vi "solar_qtimer Get Qtimer Names for Target.vi"(10 "Target Name":string, 11 "QTimers":T1[](array[typedef])) -> (3 "Target's Qtimer Names":string[](array[string]))   [LabVIEW 2018]
doc: "Outputs target names for each of the specified qtimers."
uses:
  solar_qtimer_ctl QTimer Settings.ctl
  solar_qtimer_ctl QTimer.ctl
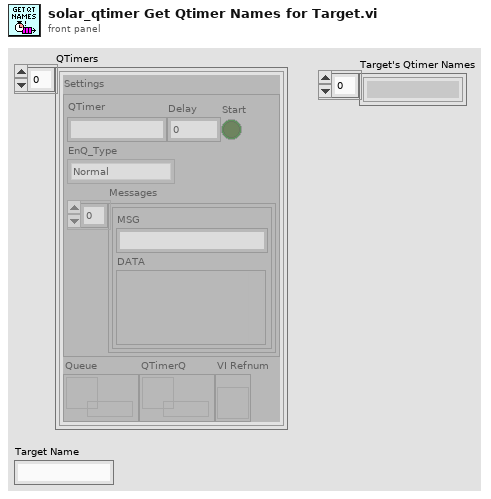
[diagram p1: front panel]
types:
  T1 = typedef "solar_qtimer_ctl QTimer.ctl" = cluster{"Settings":T2, "Queue":refnum<queue>, "QTimerQ":refnum<queue>, "VI Refnum":refnum<vi>}
  T2 = typedef "solar_qtimer_ctl QTimer Settings.ctl" = cluster{"QTimer":string, "Delay":i32, "Start":bool, "EnQ_Type":enum8{"Normal", "Priority", "IgnoreIfExists"}, "Messages":cluster{"MSG":string, "DATA":variant}[]}
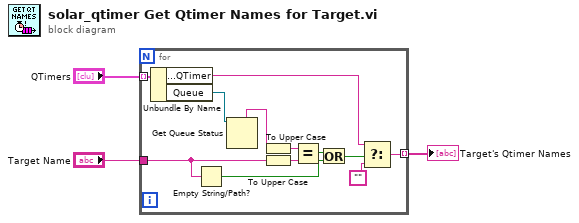
[diagram p0: block diagram]
diagram:
  n1 = for {
    tunnel: "QTimers" -> [w15] mode=indexing
    tunnel: [w7] -> w1 mode=indexing
    tunnel: "Target Name" -> [w6]
    n2 = Unbundle By Name(w15) -> ("Settings.QTimer"=w8:string, "Queue"=w14:refnum<queue>)
    n3 = Empty String/Path?(string/path=w6) -> (empty?=w4:bool)
    n4 = Get Queue Status(queue=w14) -> (queue name=w11:string)  [unwired: 2 in, 7 out]
    n5 = To Upper Case(1:w11) -> (0:w13:string)
    n6 = To Upper Case(1:w6) -> (0:w12:string)
    n7 = Equal?(x=w13, y=w12) -> (x = y?=w10:bool)
    n8 = Or(x=w10, y=w4) -> (x .or. y?=w5:bool)
    n9 = Select(t=w8, s=w5, f="") -> (s? t:f=w7:string)
  }
  "Target's Qtimer Names" <- w1
